vi "Read Dictionary.vi"(1 "Numeric":i32, 2 "Dictionary In":T1[](array[typedef])) -> (0 "data":dbl[](array[numeric]))   [LabVIEW 2020]
uses:
  <userlib>/LevyLab/LV to ITX/Data/Typedefs/Dictionary--cluster.ctl
  <userlib>/LevyLab/LV to ITX/Data/Data.lvclass
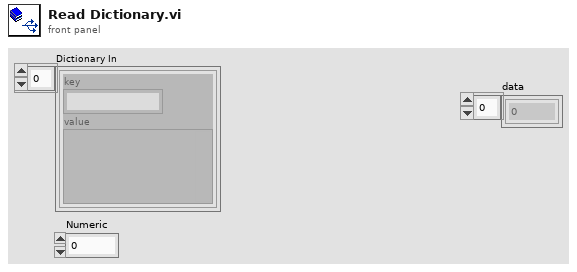
[diagram p1: front panel]
types:
  T1 = typedef "Data.lvclass/Dictionary--cluster.ctl" = cluster{"key":string, "value":variant}
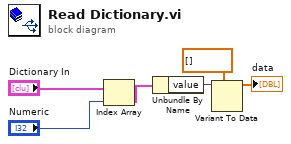
[diagram p0: block diagram]
diagram:
  n1 = Index Array(array="Dictionary In", index="Numeric") -> (element=w4:T1)
  n2 = Unbundle By Name(w4) -> ("value"=w3:variant)
  n3 = Variant To Data(type=dbl[] [], Variant=w3) -> (data=→"data":dbl[])  [unwired: 1 in, 1 out]
